vi "Traditional UI.vi"(11 "Process in":refnum<class "Process.lvclass">) -> (0 "error out":errorcluster, 3 "Process out":refnum<class "Process.lvclass">)   [LabVIEW 2021, in "Process.lvlib" / "Process.lvclass"]
uses:
  Process.lvclass
  AAM/AAM/Self Actor/Self Actor.lvclass
  Process.lvclass/Process.ctl
  AAM/Msgs/Destroy/Destroy Msg/Destroy Msg.lvclass
  C:/PPLs/LabVIEW-Composed-Actor-Model-LVCAM/LabVIEW-Composed-Actor-Model-LVCAM/AAM/AAM/Msg/Msg.lvclass
  AAM/AAM/Self Actor/Self Msg Send.vi
  C:/PPLs/LabVIEW-Composed-Actor-Model-LVCAM/LabVIEW-Composed-Actor-Model-LVCAM/AAM/Msgs/Destroy/Destroy Msg/Destroy Msg.lvclass
panel:
  # "PANEL"
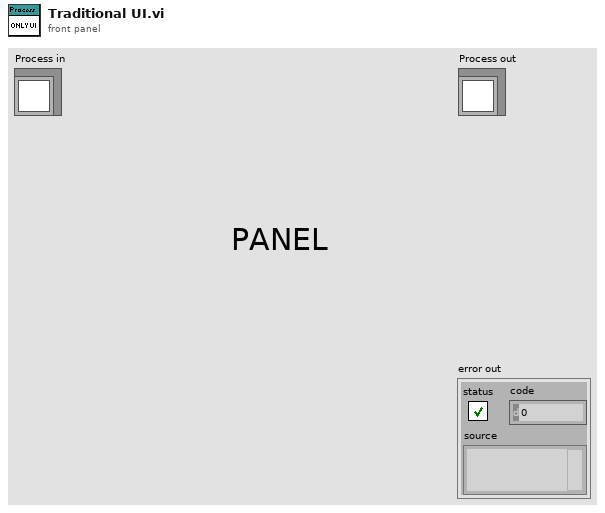
[diagram p1: front panel]
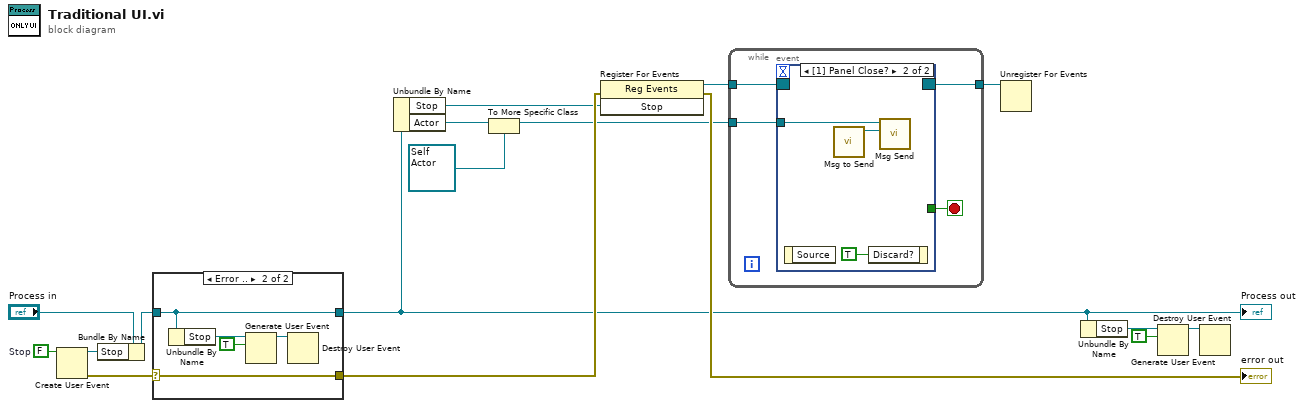
[diagram p0: block diagram]
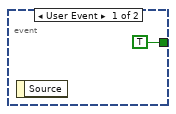
[diagram p2: hidden frame]
diagram:
  w15 = FALSE  # Stop
  n1 = Create User Event(user event datatype=w15) -> (user event=w16:refnum<user-event>, error out=w14:errorcluster)  [unwired: 1 in]
  n2 = Bundle By Name(cluster="Process in", "Stop"=w16) -> (w13:refnum<class "Process.lvclass">)
  n3 = case shown="Error .." w14 {
    selector: w14 -> [_ w23]
    tunnel: [w18 w19] -> w4
    tunnel: w13 -> [w18 w19]
    tunnel: [_ w23] -> w9
    frame No Error {
    }
    frame Error {
      n4 = Unbundle By Name(w19) -> ("Stop"=w20:refnum<user-event>)
      n5 = Generate User Event(user event=w20, event data cluster=TRUE ("event data")) -> (user event out=w21:refnum<user-event>)  [unwired: 2 in, 1 out]
      n6 = Destroy User Event(user event=w21) -> ()  [unwired: 1 in, 1 out]
    }
  }
  "Process out" <- w4
  n7 = Unbundle By Name(w4) -> ("Stop"=w8:refnum<user-event>, "Actor"=w3:refnum<class "Actor.lvclass">)
  n8 = To More Specific Class(target class=refnum<class "Self Actor.lvclass"> refnum ("AAM.lvlib:Self Actor.lvclass"), reference=w3) -> (specific class reference=w2:refnum<class "Self Actor.lvclass">)  [unwired: 1 in, 1 out]
  n9 = register-events ("Main Register for Events")(error in=w9, w8) -> (reference out=w12:refnum<event-registration>, error out=→"error out":errorcluster)  [unwired: 1 in]
  n10 = while {
    tunnel: w12 -> [w27]
    tunnel: [w25] -> w11
    tunnel: w2 -> [w24]
    stop <- w26 stop-if-true
    n11 = event "UI Events" shown="[1] Panel Close?" {
      selector: w27 -> [_ _]
      dyn-events: [_ _] -> w25
      timeout: _ -> [_ _]
      tunnel: [TRUE _] -> w26
      tunnel: w24 -> [_ w30]
      event User Event {
        n12 = event-data() -> ()  [unwired: 1 in, 1 out]
      }
      event Panel Close? {
        n13 = event-data() -> ()  [unwired: 1 in, 1 out]
        n14 = call "Msg to Send.vi"() -> ("Destroy Msg out"=w29:refnum<class "Destroy Msg.lvclass">)  [unwired: 11 in]
        n15 = event-data("Discard?"=TRUE) -> ()  [unwired: 1 in, 1 out]
        n16 = call-poly "Msg Send.vi"("Msg"=w29, "Self Actor in"=w30) -> ()  [unwired: 9 in, 1 out]
      }
    }
  }
  n17 = Unregister For Events(event registration refnum=w11) -> ()  [unwired: 1 in, 1 out]
  n18 = Unbundle By Name(w4) -> ("Stop"=w7:refnum<user-event>)
  n19 = Generate User Event(user event=w7, event data cluster=TRUE ("event data")) -> (user event out=w6:refnum<user-event>)  [unwired: 2 in, 1 out]
  n20 = Destroy User Event(user event=w6) -> ()  [unwired: 1 in, 1 out]
